vi "Example.vi"() -> ()   [LabVIEW 2016]
uses:
  System.Windows.Forms
  source code/API/MDI_Class/LV MDI.lvclass
  <vilib>/Utility/miscctls.llb/LVRectTypeDef.ctl
  source code/API/MDI_Class/Public/Create.vi
  source code/API/MDI_Class/Public/Destroy.vi
  source code/API/MDI_Class/Public/Load.vi
  source code/API/MDI_Class/Public/Set Position.vi
  source code/API/MDI_Class/Public/Add.vi
  source code/API/MDI_Class/Public/Dock.vi
  source code/API/MDI_Class/Public/Remove.vi
panel:
  in  "Listbox":i32[](listbox)
  in  "Tile":bool
  in  "Undock":bool
  in  "Load":bool
  in  "Destroy":bool
  in  "Remove":bool
  out "Error Out":errorcluster
  in  "Error in":errorcluster
  in  "ADD/Display":bool
  in  "Stop":bool
  in  "Create":bool
  in  "Vi Path":path=path "D:/MDI Project/example/Waveform.vi"
  in  "Container":refnum<k24>(container)
  # "Instructions:\n1.Select the Path and press load to load the VI.\n2.Press ADD to add vi in cointainer and display."
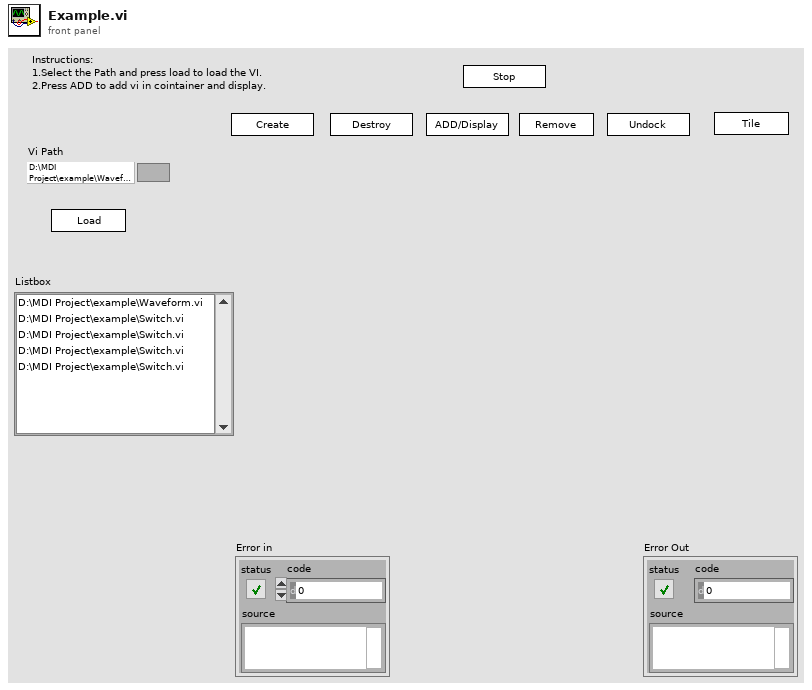
[diagram p1: front panel]
types:
  T1 = typedef "LVRectTypeDef.ctl" = cluster{"Left":i16, "Top":i16, "Right":i16, "Bottom":i16}
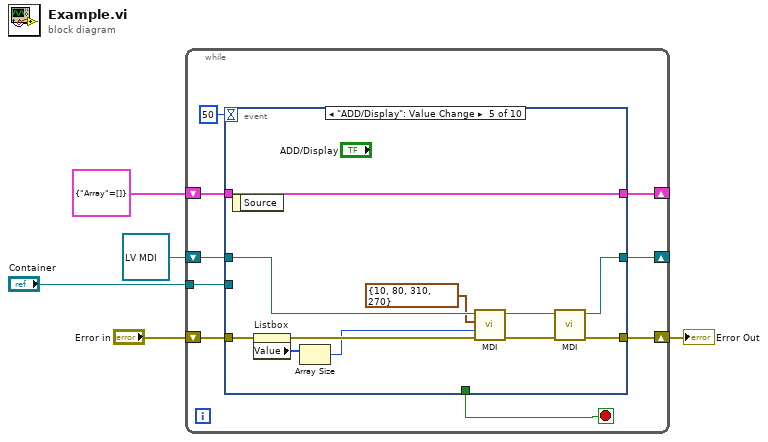
[diagram p0: block diagram]
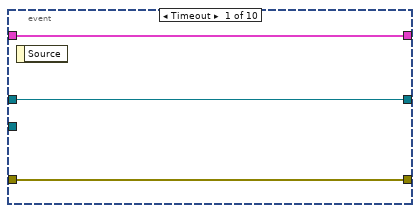
[diagram p2: hidden frame]
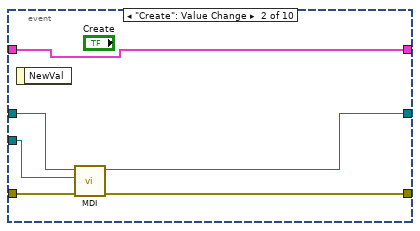
[diagram p3: hidden frame]
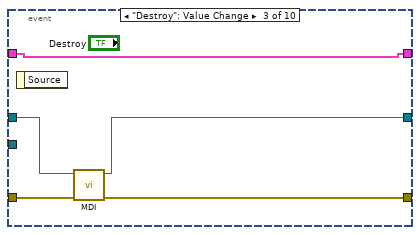
[diagram p4: hidden frame]
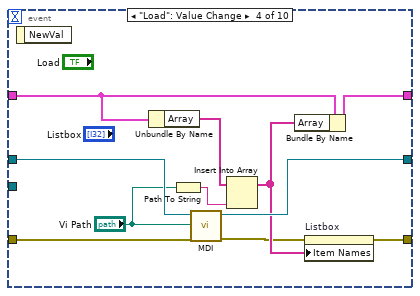
[diagram p5: hidden frame]
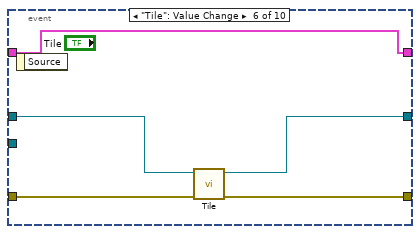
[diagram p6: hidden frame]
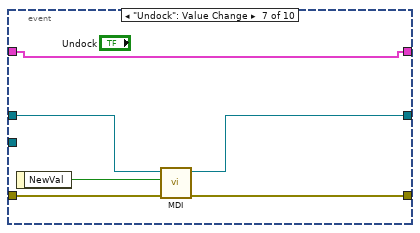
[diagram p7: hidden frame]
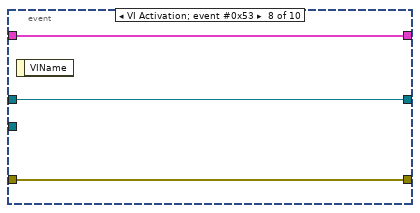
[diagram p8: hidden frame]
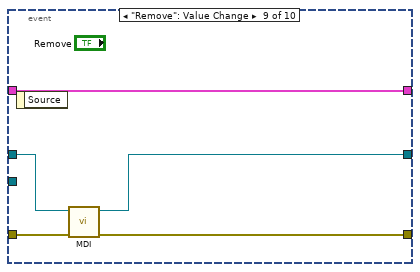
[diagram p9: hidden frame]
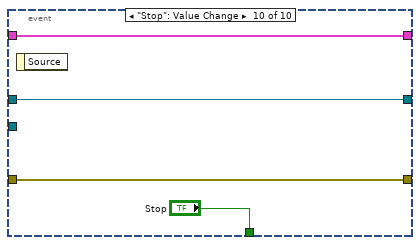
[diagram p10: hidden frame]
diagram:
  n1 = while {
    tunnel: "Container" -> [w11]
    shift-right: [w9] -> w2
    shift-left: "Error in" -> [w10]
    shift-right: [w8] -> _
    shift-left: refnum<class "LV MDI.lvclass"> refnum ("MDI.lvlib:LV MDI.lvclass") -> [w12]
    shift-right: [w6] -> _
    shift-left: cluster{"Array":string[]} {"Array"=[]} -> [w7]
    stop <- w13 stop-if-true
    n2 = event shown="[4] \"ADD/Display\": Value Change" {
      selector: _ -> [_ _ _ _ _ _ _ _ _ _]
      dyn-events: _ -> [_ _ _ _ _ _ _ _ _ _]
      timeout: 50 -> [_ _ _ _ _ _ _ _ _ _]
      tunnel: [_ _ _ _ _ _ _ _ _ "Stop"] -> w13
      tunnel: w12 -> [w16 w23 w27 w38 w46 w53 w59 w63 w67 w71]
      tunnel: w11 -> [_ w22 _ _ _ _ _ _ _ _]
      tunnel: w10 -> [w17 w20 w28 w39 w43 w55 w61 w64 w69 w72]
      tunnel: [w17 w19 w25 w29 w49 w54 w60 w64 w68 w72] -> w9
      tunnel: [w16 w21 w26 w37 w47 w52 w58 w63 w66 w71] -> w8
      tunnel: w7 -> [w15 w18 w24 w34 w45 w51 w56 w62 w65 w70]
      tunnel: [w15 w18 w24 w33 w45 w51 w56 w62 w65 w70] -> w6
      event Timeout {
        n3 = event-data() -> ()  [unwired: 1 in, 1 out]
      }
      event "Create": Value Change {
        n4 = event-data() -> ()  [unwired: 1 in, 1 out]
        n5 = call-poly "MDI.vi"("error in (no error)"=w20, "Panel"=w22, "LV MDI in"=w23) -> ("error out"=w19:errorcluster, "LV MDI out"=w21:refnum<class "LV MDI.lvclass">)  [unwired: 7 in]
      }
      event "Destroy": Value Change {
        n6 = event-data() -> ()  [unwired: 1 in, 1 out]
        n7 = call-poly "MDI.vi"("error in (no error)"=w28, "LV MDI in"=w27) -> ("error out"=w25:errorcluster, "LV MDI out"=w26:refnum<class "LV MDI.lvclass">)  [unwired: 8 in]
      }
      event "Load": Value Change {
        n8 = event-data() -> ()  [unwired: 1 in, 1 out]
        n9 = Unbundle By Name(w34) -> ("Array"=w32:string[])
        n10 = Path To String(path="Vi Path") -> (string=w31:string)
        n11 = call-poly "MDI.vi"("error in (no error)"=w39, "Vi Path"="Vi Path", "LV MDI in"=w38) -> ("error out"=w30:errorcluster, "LV MDI out"=w37:refnum<class "LV MDI.lvclass">)  [unwired: 6 in, 1 out]
        n12 = Insert Into Array(array=w32, new element=w31) -> (w35:string[])  [unwired: 1 in]
        n13 = Bundle By Name(cluster=w34, "Array"=w35) -> (w33:cluster{"Array":string[]})
        n14 = property on="Listbox" class="LstBox (strict)"(error in=w30, "Item Names"=w35) -> (error out=w29:errorcluster)  [unwired: 1 in, 1 out]
      }
      event "ADD/Display": Value Change {
        n15 = event-data() -> ()  [unwired: 1 in, 1 out]
        n16 = property on="Listbox" class="LstBox (strict)"(error in=w43) -> (error out=w42:errorcluster, "Value"=w44:i32[])  [unwired: 1 in, 1 out]
        n17 = Array Size(array=w44) -> (size(s)=w41:i32)
        n18 = call-poly "MDI.vi"("error in (no error)"=w42, "Increment"=w41, "FP Bounds"=T1 {"Left"=10, "Top"=80, "Right"=310, "Bottom"=270}, "LV MDI.lvclass"=w46) -> ("error out"=w50:errorcluster, "LV MDI.lvclass"=w48:refnum<class "LV MDI.lvclass">)  [unwired: 6 in]
        n19 = call-poly "MDI.vi"("error in (no error)"=w50, "LV MDI in"=w48) -> ("error out"=w49:errorcluster, "LV MDI out"=w47:refnum<class "LV MDI.lvclass">)  [unwired: 8 in]
      }
      event "Tile": Value Change {
        n20 = event-data() -> ()  [unwired: 1 in, 1 out]
        n21 = call "Tile.vi"("error in (no error)"=w55, "LV MDI.lvclass"=w53) -> ("error out"=w54:errorcluster, "LV MDI.lvclass"=w52:refnum<class "LV MDI.lvclass">)  [unwired: 8 in]
      }
      event "Undock": Value Change {
        n22 = event-data() -> ("NewVal"=w57:bool)  [unwired: 1 in]
        n23 = call-poly "MDI.vi"("error in (no error)"=w61, "Undock?"=w57, "LV MDI.lvclass"=w59) -> ("error out"=w60:errorcluster, "LV MDI.lvclass"=w58:refnum<class "LV MDI.lvclass">)  [unwired: 7 in]
      }
      event VI Activation; event #0x53 {
        n24 = event-data() -> ()  [unwired: 1 in, 1 out]
      }
      event "Remove": Value Change {
        n25 = event-data() -> ()  [unwired: 1 in, 1 out]
        n26 = call-poly "MDI.vi"("error in (no error)"=w69, "LV MDI in"=w67) -> ("error out"=w68:errorcluster, "LV MDI out"=w66:refnum<class "LV MDI.lvclass">)  [unwired: 8 in]
      }
      event "Stop": Value Change {
        n27 = event-data() -> ()  [unwired: 1 in, 1 out]
      }
    }
  }
  "Error Out" <- w2
